vi "Main.vi"(11 "Module Admin":refnum<class "Delacor_lib_QMH_Cloneable Module Admin.lvclass">) -> ()   [LabVIEW 2020, in "NI DAQ Aug 25.lvlib"]
doc: "This template is based off of the Queued Message Handler design pattern and the Queued Message Handler project template that ships with LabVIEW.\n\nThe main difference is that the queue is private to this module and communication between modules is performed via Broadcast and Request events.\n\nRequest events are wrapped in public API methods and are handled in the Event Handling Loop (EHL) of this VI. Any module can register for Broadcast events sent by this module. The EHL generates messages based on user interface actions.\n\nThe Message Handling Loop (MHL) processes messages generated by the EHL, or by other messages. The messages are string values, so new messages can be added easily to the Message Cases case structure in the MHL. Each message cluster can also provide an optional value for Message Data, which is a variant that can be converted to whatever message-specific data is required.\n_____\nBased on DQMH Dev Tools: Project Template 7.1.0.1499."
uses:
  NI DAQ Aug 25.lvlib
  <vilib>/Delacor/Delacor QMH/Libraries/Cloneable Module Admin_class/Delacor_lib_QMH_Cloneable Module Admin.lvclass
  C:/Program Files (x86)/National Instruments/LabVIEW 2025/vi.lib/Delacor/Delacor QMH/Libraries/Module Admin_class/Delacor_lib_QMH_Module Admin.lvclass
  <vilib>/Delacor/Delacor QMH/Libraries/Message Queue_class/Delacor_lib_QMH_Message Queue.lvclass/Delacor_lib_QMH_Message Queue.ctl
  <vilib>/Delacor/Delacor QMH/Libraries/Cloneable Module Admin_class/Delacor_lib_QMH_Cloneable Module Admin.lvclass/Delacor_lib_QMH_Cloneable Module Admin.ctl
  <vilib>/Delacor/Delacor QMH/Libraries/Module Admin_class/Delacor_lib_QMH_Module Admin.lvclass/Delacor_lib_QMH_Module Admin.ctl
  <vilib>/Delacor/Delacor QMH/Libraries/Message Queue_class/Delacor_lib_QMH_Message Queue.lvclass
  Module Data--cluster.ctl
  <vilib>/Utility/miscctls.llb/LVPointTypeDef.ctl
  <vilib>/Delacor/Delacor QMH/Libraries/Message Queue_class/Delacor_lib_QMH_Enqueue Message (Single).vi
  Stop Argument--cluster.ctl
  Draw FP in subpanel Argument--cluster.ctl
  Remove from subpanel Argument--cluster.ctl
  Set device name Argument--cluster.ctl
  <resource>/objmgr/daqmx.rc
  Ports --typedef.ctl
  Write DO Argument--cluster.ctl
  Create DO channel Argument--cluster.ctl
  <vilib>/DAQmx/create/channels.llb/DAQmx Create Channel (DO-Digital Output).vi
  Acquisition type--typedef.ctl
  <vilib>/DAQmx/write.llb/DAQmx Write (Digital Bool 1Line 1Point).vi
  <vilib>/DAQmx/write.llb/DAQmx Write (Digital 1D U8 1Chan NSamp).vi
panel:
  out "error out":errorcluster
  out "Status":string
  in  "Simulate EHL Error":bool
  in  "Simulate MHL Error":bool
  # "Other processes communicate with this Module via its Public API (wrappers for its Request Events).\n\nThis Module communicates with other processes via its Broadcast Events.\nAny process that wants to receive these messages can register for this module's Broadcast events."
  # "This template is for the DQMH framework. See the block diagram for more information on how to use this template."
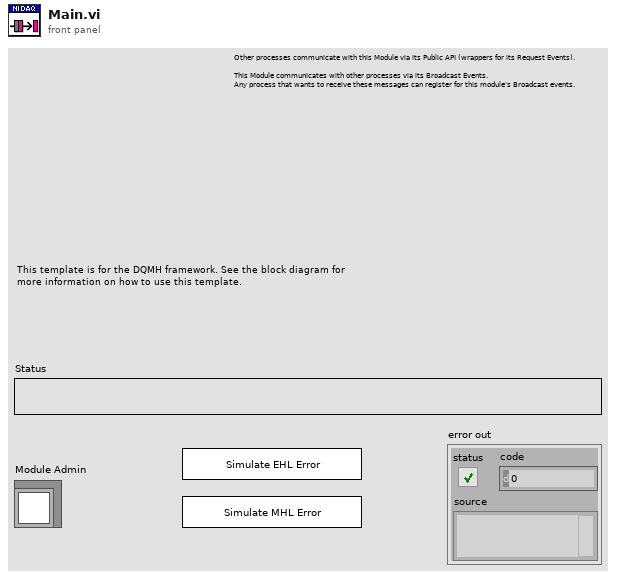
[diagram p1: front panel]
types:
  T1 = typedef "NI DAQ Aug 25.lvlib/Request Events--cluster.ctl" = cluster{"Stop Module":refnum<user-event>, "Show Panel":refnum<user-event>, "Hide Panel":refnum<user-event>, "Show Diagram":refnum<user-event>, "Get Module Execution Status":refnum<user-event>, "Draw FP in subpanel":refnum<user-event>, "Remove from subpanel":refnum<user-event>, "Set device name":refnum<user-event>, "Write DO":refnum<user-event>, "Create DO channel":refnum<user-event>}
  T2 = typedef "NI DAQ Aug 25.lvlib/Module Data--cluster.ctl" = cluster{"Status":string, "Sub Panel":refnum<vi>, "Device Name":tag, "Is simulated?":bool, "DO channel":refnum<k21>}
  T3 = enum32{"invalid lock state", "Not Locked", "Locked (No Password)", "Password-protected"}
  T4 = typedef "NI DAQ Aug 25.lvlib/Stop Argument--cluster.ctl" = cluster{"Module ID":i32, "Origin":string, "Exit via Stop Module Req?":bool, "Wait for Module to stop?":bool}
  T5 = typedef "NI DAQ Aug 25.lvlib/Draw FP in subpanel Argument--cluster.ctl" = cluster{"Module ID":i32, "Sub Panel":refnum<vi>}
  T6 = typedef "NI DAQ Aug 25.lvlib/Remove from subpanel Argument--cluster.ctl" = cluster{"Module ID":i32, "Boolean":bool}
  T7 = typedef "NI DAQ Aug 25.lvlib/Set device name Argument--cluster.ctl" = cluster{"Module ID":i32, "DAQmx Device Name":tag}
  T8 = typedef "NI DAQ Aug 25.lvlib/Write DO Argument--cluster.ctl" = cluster{"Module ID":i32, "Port":T9, "DO":bool[], "Acq type":T10}
  T9 = typedef "Ports --typedef.ctl" = enum16{"port0", "port1"}
  T10 = typedef "Acquisition type--typedef.ctl" = enum16{"Single", "Multiple"}
  T11 = typedef "NI DAQ Aug 25.lvlib/Create DO channel Argument--cluster.ctl" = cluster{"Module ID":i32, "Port":T9, "Lines":string}
  T12 = typedef "LVPointTypeDef.ctl" = cluster{"Horizontal":i16, "Vertical":i16}
  T13 = enum32{"Invalid", "Standard", "Closed", "Hidden", "Minimized", "Maximized"}
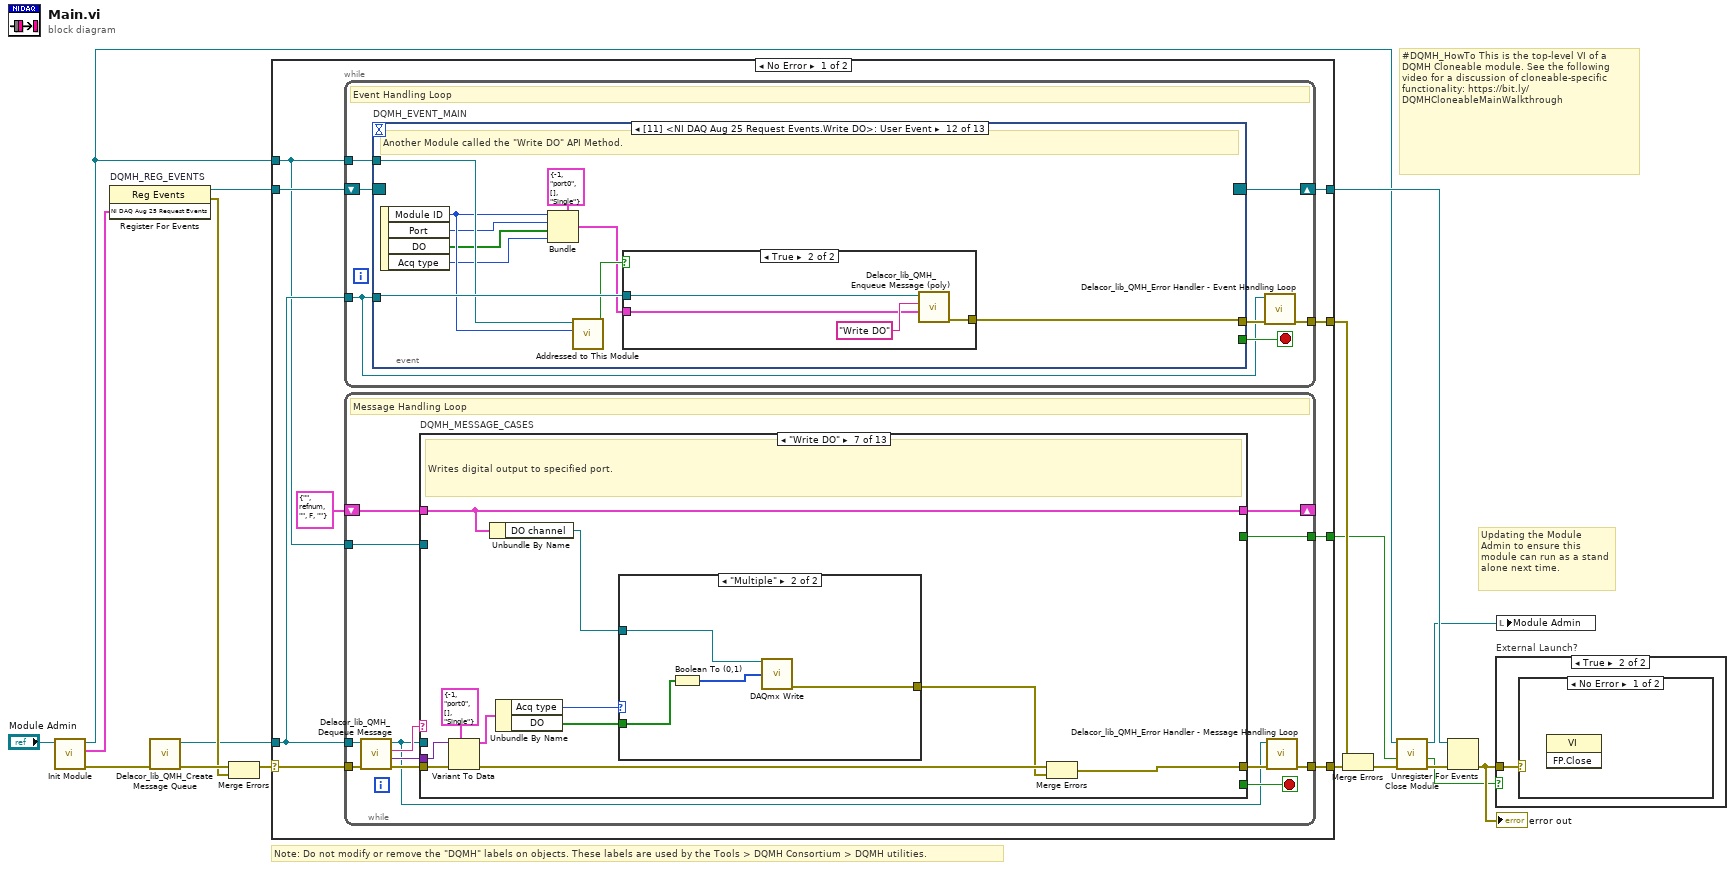
[diagram p0: block diagram]
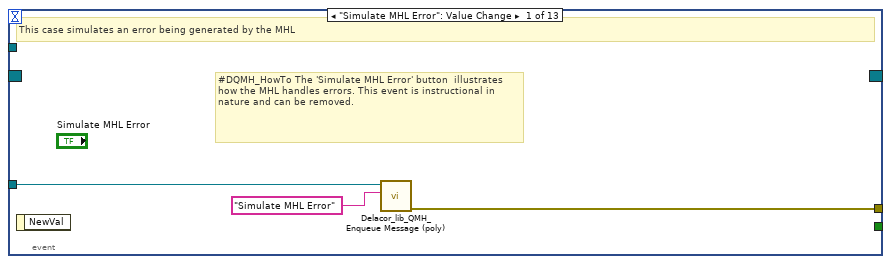
[diagram p2: hidden frame]
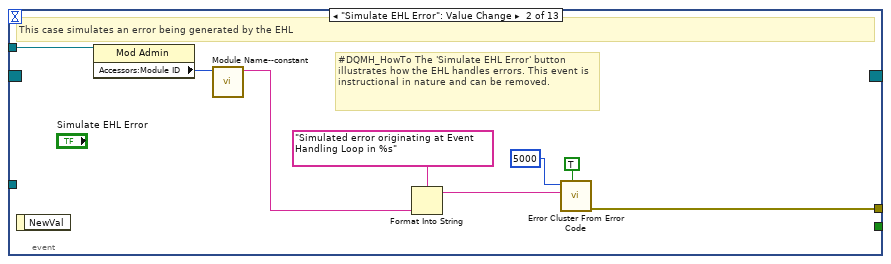
[diagram p3: hidden frame]
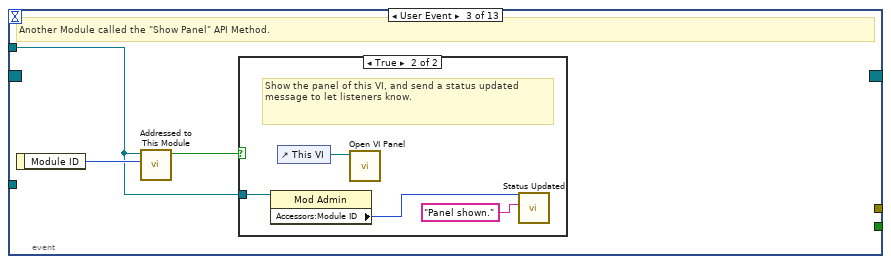
[diagram p4: hidden frame]
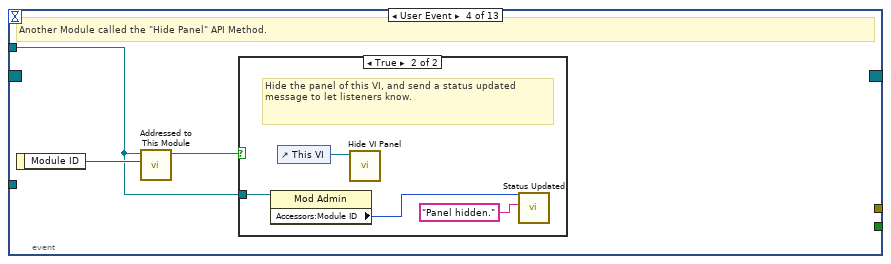
[diagram p6: hidden frame]
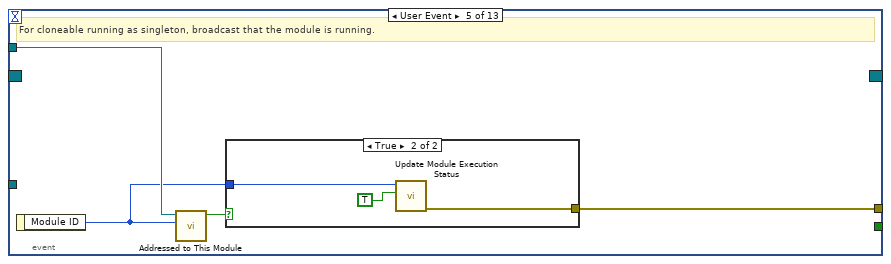
[diagram p8: hidden frame]
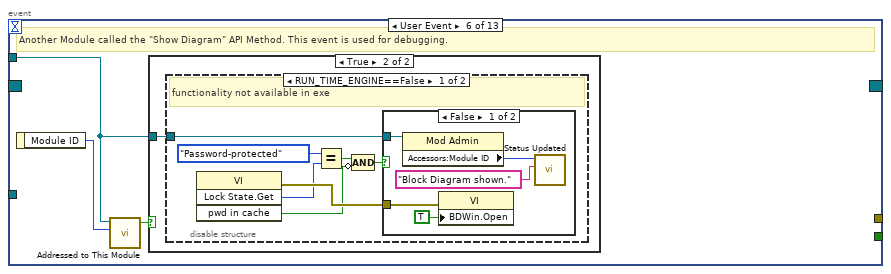
[diagram p10: hidden frame]
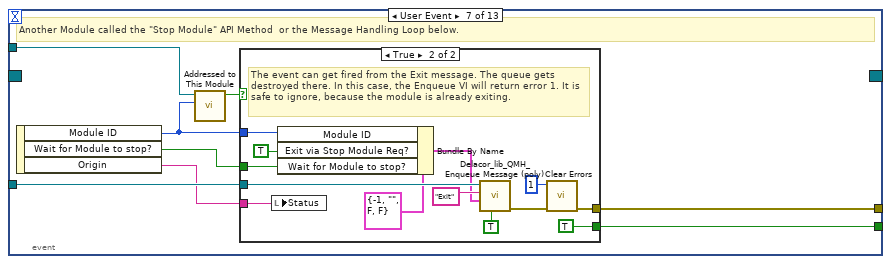
[diagram p14: hidden frame]
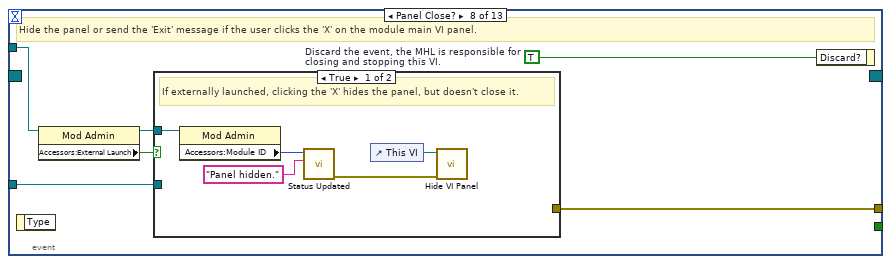
[diagram p16: hidden frame]
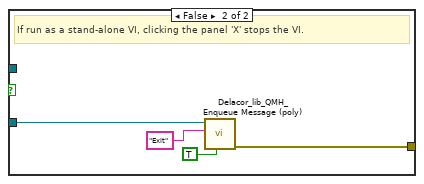
[diagram p17: hidden frame]
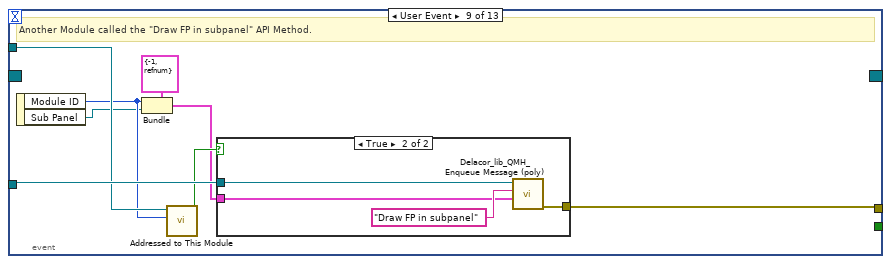
[diagram p18: hidden frame]
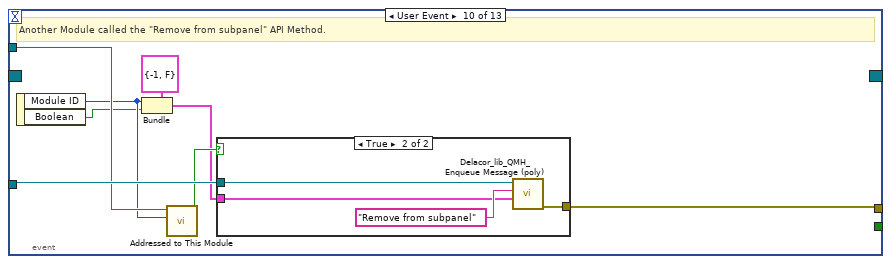
[diagram p20: hidden frame]
diagram:
  # "#DQMH_HowTo This is the top-level VI of a DQMH Cloneable module. See the following video for a discussion of cloneable-specific functionality: https://bit.ly/DQMHCloneableMainWalkthrough"
  # "Note: Do not modify or remove the \"DQMH\" labels on objects. These labels are used by the Tools > DQMH Consortium > DQMH utilities."
  # "Updating the Module Admin to ensure this module can run as a stand alone next time."
  n1 = call "Init Module.vi"("Cloneable Module Admin in"="Module Admin") -> ("error out"=w15:errorcluster, "NI DAQ Aug 25 Request Events"=w7:T1, "Cloneable Module Admin out"=w4:refnum<class "Delacor_lib_QMH_Cloneable Module Admin.lvclass">)  [unwired: 8 in]
  n2 = register-events "DQMH_REG_EVENTS"(w7) -> (reference out=w8:refnum<event-registration>, error out=w10:errorcluster)  [unwired: 2 in]
  n3 = call <vilib>:"Delacor_lib_QMH_Create Message Queue.vi"("error in"=w15) -> ("error out"=w12:errorcluster, "Message Queue"=w6:refnum<class "Delacor_lib_QMH_Message Queue.lvclass">)  [unwired: 9 in]
  n4 = Merge Errors(w12, w10) -> (w11:errorcluster)
  n5 = case shown="No Error" w11 {
    selector: w11 -> [w25 w377]
    tunnel: [w27 w376] -> w16
    tunnel: [w24 w375] -> w9
    tunnel: w8 -> [w22 w375]
    tunnel: w6 -> [w21 w368]
    tunnel: [w26 _] -> w17
    tunnel: w4 -> [w20 w371]
    tunnel: [w19 _] -> w2
    frame No Error {
      n6 = while {
        tunnel: w21 -> [w28]
        shift-right: [w31] -> w24
        shift-left: w22 -> [w32]
        tunnel: [w33] -> w26
        tunnel: w20 -> [w29]
        stop <- w30 stop-if-true
        # "Event Handling Loop"
        n7 = event "DQMH_EVENT_MAIN" shown="[11] <NI DAQ Aug 25 Request Events.Write DO>: User Event" {
          selector: w32 -> [_ _ _ _ _ _ _ _ _ _ _ _ _]
          dyn-events: [_ _ _ _ _ _ _ _ _ _ _ _ _] -> w31
          timeout: _ -> [_ _ _ _ _ _ _ _ _ _ _ _ _]
          tunnel: [_ _ _ _ _ _ w86 _ _ _ _ _ _] -> w30
          tunnel: w28 -> [w36 _ _ _ _ _ w89 w106 w126 w138 w150 w164 w177]
          tunnel: [w37 w45 _ _ w63 _ w90 w109 w119 w131 w143 w156 w169] -> w34
          tunnel: w29 -> [_ w44 w46 w53 w61 w67 w88 w107 w124 w136 w148 w162 w175]
          event "Simulate MHL Error": Value Change {
            # "#DQMH_HowTo The 'Simulate MHL Error' button  illustrates how the MHL handles errors. This event is instructional in nature and can be removed."
            # "This case simulates an error being generated by the MHL"
            n8 = event-data() -> ()  [unwired: 1 in, 1 out]
            n9 = call-poly <vilib>:"Delacor_lib_QMH_Enqueue Message (poly).vi"("Message"="Simulate MHL Error", "Message Queue in"=w36) -> ("error out"=w37:errorcluster)  [unwired: 8 in, 1 out]
          }
          event "Simulate EHL Error": Value Change {
            # "#DQMH_HowTo The 'Simulate EHL Error' button  illustrates how the EHL handles errors. This event is instructional in nature and can be removed."
            # "This case simulates an error being generated by the EHL"
            n10 = event-data() -> ()  [unwired: 1 in, 1 out]
            n11 = property on="Property Node" class="Mod Admin"(reference=w44) -> ("Accessors:Module ID"=w43:i32)  [unwired: 1 in, 2 out]
            n12 = call "Module Name--constant.vi"("Module ID"=w43) -> ("Module Name"=w38:string)  [unwired: 10 in]
            n13 = Format Into String(format string="Simulated error originating at Event Handling Loop in %s", w38) -> (resulting string=w41:string)  [unwired: 2 in, 1 out]
            n14 = call <vilib>:"Error Cluster From Error Code.vi"("show call chain? (False)"=TRUE, "error message (\"\")"=w41, "error code (0)"=5000) -> ("error out"=w45:errorcluster)  [unwired: 6 in]
          }
          event User Event {
            # "Another Module called the \"Show Panel\" API Method."
            n15 = event-data() -> ("Module ID"=w47:i32)  [unwired: 1 in]
            n16 = call "Addressed to This Module.vi"("Module ID from Argument"=w47, "Module Admin"=w46) -> ("Addressed to this instance?"=w48:bool)  [unwired: 8 in, 1 out]
            n17 = case shown="True" w48 {
              tunnel: w46 -> [_ w50]
              frame False {
              }
              frame True {
                # "Show the panel of this VI, and send a status updated message to let listeners know."
                n18 = property on="Property Node" class="Mod Admin"(reference=w50) -> ("Accessors:Module ID"=w49:i32)  [unwired: 1 in, 2 out]
                n19 = control-ref of="This VI"() -> (w52:refnum<vi>)
                n20 = call "Open VI Panel.vi"("VI"=w52) -> ()  [unwired: 10 in, 1 out]
                n21 = call "Status Updated.vi"("Status"="Panel shown." ("format string"), "Module ID"=w49) -> ()  [unwired: 9 in, 1 out]
              }
            }
          }
          event User Event {
            # "Another Module called the \"Hide Panel\" API Method."
            n22 = event-data() -> ("Module ID"=w54:i32)  [unwired: 1 in]
            n23 = call "Addressed to This Module.vi"("Module ID from Argument"=w54, "Module Admin"=w53) -> ("Addressed to this instance?"=w55:bool)  [unwired: 8 in, 1 out]
            n24 = case shown="True" w55 {
              tunnel: w53 -> [_ w57]
              frame False {
              }
              frame True {
                # "Hide the panel of this VI, and send a status updated message to let listeners know."
                n25 = property on="Property Node" class="Mod Admin"(reference=w57) -> ("Accessors:Module ID"=w56:i32)  [unwired: 1 in, 2 out]
                n26 = control-ref of="This VI"() -> (w59:refnum<vi>)
                n27 = call "Hide VI Panel.vi"("VI"=w59) -> ()  [unwired: 10 in, 1 out]
                n28 = call "Status Updated.vi"("Status"="Panel hidden." ("format string"), "Module ID"=w56) -> ()  [unwired: 9 in, 1 out]
              }
            }
          }
          event User Event {
            # "For cloneable running as singleton, broadcast that the module is running."
            n29 = event-data() -> ("Module ID"=w60:i32)  [unwired: 1 in]
            n30 = call "Addressed to This Module.vi"("Module ID from Argument"=w60, "Module Admin"=w61) -> ("Addressed to this instance?"=w62:bool)  [unwired: 8 in, 1 out]
            n31 = case shown="True" w62 {
              tunnel: [_ w66] -> w63
              tunnel: w60 -> [_ w65]
              frame False {
              }
              frame True {
                n32 = call "Update Module Execution Status.vi"("Running?"=TRUE, "Module ID"=w65) -> ("error out"=w66:errorcluster)  [unwired: 9 in]
              }
            }
          }
          event User Event {
            # "Another Module called the \"Show Diagram\" API Method. This event is used for debugging."
            n33 = event-data() -> ("Module ID"=w68:i32)  [unwired: 1 in]
            n34 = call "Addressed to This Module.vi"("Module ID from Argument"=w68, "Module Admin"=w67) -> ("Addressed to this instance?"=w69:bool)  [unwired: 8 in, 1 out]
            n35 = case shown="True" w69 {
              tunnel: w67 -> [_ w70]
              frame False {
              }
              frame True {
                n36 = disable-structure shown="RUN_TIME_ENGINE==False" {
                  disable-tunnel: w70 -> [w71 _]
                  frame condition #0 (active) {
                    # "functionality not available in exe"
                    n37 = invoke on="Invoke Node" class="VI" method="Lock State.Get"() -> (error out=w77:errorcluster, "Get Lock State"=w76:T3, "pwd in cache"=w73:bool)  [unwired: 4 in, 1 out]
                    n38 = Equal?(x=T3."Password-protected", y=w76) -> (x = y?=w74:bool)
                    n39 = Compound Arithmetic op=AND(w74, invert w73) -> (w72:bool)
                    n40 = case shown="False" w72 {
                      tunnel: w77 -> [w82 _]
                      tunnel: w71 -> [w79 _]
                      frame False {
                        n41 = property on="Property Node" class="Mod Admin"(reference=w79) -> ("Accessors:Module ID"=w78:i32)  [unwired: 1 in, 2 out]
                        n42 = property on="Property Node" class="VI"(error in=w82, "BDWin.Open"=TRUE ("Block Diagram Window:Open")) -> ()  [unwired: 1 in, 2 out]
                        n43 = call "Status Updated.vi"("Status"="Block Diagram shown." ("format string"), "Module ID"=w78) -> ()  [unwired: 9 in, 1 out]
                      }
                      frame True {
                        # "Password-protected VI, and the password is not in the cache. Do not show the diagram."
                      }
                    }
                  }
                  frame condition #1 {
                  }
                }
              }
            }
          }
          event User Event {
            # "Another Module called the \"Stop Module\" API Method  or the Message Handling Loop below."
            n44 = event-data() -> ("Module ID"=w84:i32, "Wait for Module to stop?"=w85:bool, "Origin"=w83:string)  [unwired: 1 in]
            n45 = call "Addressed to This Module.vi"("Module ID from Argument"=w84, "Module Admin"=w88) -> ("Addressed to this instance?"=w87:bool)  [unwired: 8 in, 1 out]
            n46 = case shown="True" w87 {
              tunnel: [_ w102] -> w90
              tunnel: w89 -> [_ w98]
              tunnel: [_ TRUE] -> w86
              tunnel: w85 -> [_ w93]
              tunnel: w84 -> [_ w95]
              tunnel: w83 -> [_ w91]
              frame False {
              }
              frame True {
                # "The event can get fired from the Exit message. The queue gets destroyed there. In this case, the Enqueue VI will return error 1. It is safe to ignore, because the module is already exiting."
                n47 = local write "Status"(w91) -> ()
                n48 = Bundle By Name(cluster=T4 {"Module ID"=-1, "Origin"="", "Exit via Stop Module Req?"=FALSE, "Wait for Module to stop?"=FALSE} ("Stop Argument"), "Module ID"=w95, "Exit via Stop Module Req?"=TRUE, "Wait for Module to stop?"=w93) -> (w92:T4)
                n49 = call-poly <vilib>:"Delacor_lib_QMH_Enqueue Message (poly).vi"("Priority Message? (F)"=TRUE, "Message Data"=w92, "Message"="Exit", "Message Queue in"=w98) -> ("error out"=w103:errorcluster)  [unwired: 6 in, 1 out]
                n50 = call <vilib>:"Clear Errors.vi"("error in (no error)"=w103, "specific error code to clear (0: all)"=1) -> ("error out"=w102:errorcluster)  [unwired: 4 in, 1 out]
              }
            }
          }
          event Panel Close? {
            w108 = TRUE  # Discard the event, the MHL is responsible for closing and stopping this VI.
            # "Hide the panel or send the 'Exit' message if the user clicks the 'X' on the module main VI panel."
            n51 = event-data() -> ()  [unwired: 1 in, 1 out]
            n52 = property on="Property Node" class="Mod Admin"(reference=w107) -> (reference out=w104:refnum<class "Delacor_lib_QMH_Cloneable Module Admin.lvclass">, "Accessors:External Launch"=w105:bool)  [unwired: 1 in, 1 out]
            n53 = case shown="True" w105 {
              tunnel: w106 -> [_ w117]
              tunnel: [_ w118] -> w109
              tunnel: w104 -> [w112 _]
              frame True {
                # "If externally launched, clicking the 'X' hides the panel, but doesn't close it."
                n54 = property on="Property Node" class="Mod Admin"(reference=w112) -> ("Accessors:Module ID"=w111:i32)  [unwired: 1 in, 2 out]
                n55 = call "Status Updated.vi"("Status"="Panel hidden." ("format string"), "Module ID"=w111) -> ("error out"=w110:errorcluster)  [unwired: 9 in]
                n56 = control-ref of="This VI"() -> (w114:refnum<vi>)
                n57 = call "Hide VI Panel.vi"("error in"=w110, "VI"=w114) -> ()  [unwired: 9 in, 1 out]
              }
              frame False {
                # "If run as a stand-alone VI, clicking the panel 'X' stops the VI."
                n58 = call-poly <vilib>:"Delacor_lib_QMH_Enqueue Message (poly).vi"("Priority Message? (F)"=TRUE, "Message"="Exit", "Message Queue in"=w117) -> ("error out"=w118:errorcluster)  [unwired: 7 in, 1 out]
              }
            }
            n59 = event-data ("Event Filter Node")("Discard?"=w108) -> ()  [unwired: 1 in, 1 out]
          }
          event User Event {
            # "Another Module called the \"Draw FP in subpanel\" API Method."
            n60 = event-data() -> ("Module ID"=w121:i32, "Sub Panel"=w120:refnum<vi>)  [unwired: 1 in]
            n61 = Bundle(cluster=T5 {"Module ID"=-1, "Sub Panel"=refnum} ("Draw FP in subpanel Argument"), "Module ID"=w121, "Sub Panel"=w120) -> (w122:T5)
            n62 = call "Addressed to This Module.vi"("Module ID from Argument"=w121, "Module Admin"=w124) -> ("Addressed to this instance?"=w125:bool)  [unwired: 8 in, 1 out]
            n63 = case shown="True" w125 {
              tunnel: w126 -> [_ w130]
              tunnel: w122 -> [_ w128]
              tunnel: [_ w127] -> w119
              frame False {
              }
              frame True {
                n64 = call-poly <vilib>:"Delacor_lib_QMH_Enqueue Message (poly).vi"("Message Data"=w128, "Message"="Draw FP in subpanel", "Message Queue in"=w130) -> ("error out"=w127:errorcluster)  [unwired: 7 in, 1 out]
              }
            }
          }
          event User Event {
            # "Another Module called the \"Remove from subpanel\" API Method."
            n65 = event-data() -> ("Module ID"=w133:i32, "Boolean"=w132:bool)  [unwired: 1 in]
            n66 = Bundle(cluster=T6 {"Module ID"=-1, "Boolean"=FALSE} ("Remove from subpanel Argument"), "Module ID"=w133, "Boolean"=w132) -> (w134:T6)
            n67 = call "Addressed to This Module.vi"("Module ID from Argument"=w133, "Module Admin"=w136) -> ("Addressed to this instance?"=w137:bool)  [unwired: 8 in, 1 out]
            n68 = case shown="True" w137 {
              tunnel: w138 -> [_ w142]
              tunnel: w134 -> [_ w140]
              tunnel: [_ w139] -> w131
              frame False {
              }
              frame True {
                n69 = call-poly <vilib>:"Delacor_lib_QMH_Enqueue Message (poly).vi"("Message Data"=w140, "Message"="Remove from subpanel", "Message Queue in"=w142) -> ("error out"=w139:errorcluster)  [unwired: 7 in, 1 out]
              }
            }
          }
          event User Event {
            # "Another Module called the \"Set device name\" API Method."
            n70 = event-data() -> ("Module ID"=w145:i32, "DAQmx Device Name"=w144:tag)  [unwired: 1 in]
            n71 = Bundle(cluster=T7 {"Module ID"=-1, "DAQmx Device Name"=""} ("Set device name Argument"), "Module ID"=w145, "DAQmx Device Name"=w144) -> (w146:T7)
            n72 = call "Addressed to This Module.vi"("Module ID from Argument"=w145, "Module Admin"=w148) -> ("Addressed to this instance?"=w149:bool)  [unwired: 8 in, 1 out]
            n73 = case shown="True" w149 {
              tunnel: w150 -> [_ w154]
              tunnel: w146 -> [_ w152]
              tunnel: [_ w151] -> w143
              frame False {
              }
              frame True {
                n74 = call-poly <vilib>:"Delacor_lib_QMH_Enqueue Message (poly).vi"("Message Data"=w152, "Message"="Set device name", "Message Queue in"=w154) -> ("error out"=w151:errorcluster)  [unwired: 7 in, 1 out]
              }
            }
          }
          event User Event {
            # "Another Module called the \"Write DO\" API Method."
            n75 = event-data() -> ("Module ID"=w159:i32, "Port"=w158:T9, "DO"=w157:bool[], "Acq type"=w155:T10)  [unwired: 1 in]
            n76 = Bundle(cluster=T8 {"Module ID"=-1, "Port"=enum."port0", "DO"=[], "Acq type"=enum."Single"} ("Write DO Argument"), "Module ID"=w159, "Port"=w158, "DO"=w157, "Acq type"=w155) -> (w160:T8)
            n77 = call "Addressed to This Module.vi"("Module ID from Argument"=w159, "Module Admin"=w162) -> ("Addressed to this instance?"=w163:bool)  [unwired: 8 in, 1 out]
            n78 = case shown="True" w163 {
              tunnel: w164 -> [_ w168]
              tunnel: w160 -> [_ w166]
              tunnel: [_ w165] -> w156
              frame False {
              }
              frame True {
                n79 = call-poly <vilib>:"Delacor_lib_QMH_Enqueue Message (poly).vi"("Message Data"=w166, "Message"="Write DO", "Message Queue in"=w168) -> ("error out"=w165:errorcluster)  [unwired: 7 in, 1 out]
              }
            }
          }
          event User Event {
            # "Another Module called the \"Create DO channel\" API Method."
            n80 = event-data() -> ("Module ID"=w172:i32, "Port"=w171:T9, "Lines"=w170:string)  [unwired: 1 in]
            n81 = Bundle(cluster=T11 {"Module ID"=-1, "Port"=enum."port0", "Lines"=""} ("Create DO channel Argument"), "Module ID"=w172, "Port"=w171, "Lines"=w170) -> (w173:T11)
            n82 = call "Addressed to This Module.vi"("Module ID from Argument"=w172, "Module Admin"=w175) -> ("Addressed to this instance?"=w176:bool)  [unwired: 8 in, 1 out]
            n83 = case shown="True" w176 {
              tunnel: w177 -> [_ w181]
              tunnel: w173 -> [_ w179]
              tunnel: [_ w178] -> w169
              frame False {
              }
              frame True {
                n84 = call-poly <vilib>:"Delacor_lib_QMH_Enqueue Message (poly).vi"("Message Data"=w179, "Message"="Create DO channel", "Message Queue in"=w181) -> ("error out"=w178:errorcluster)  [unwired: 7 in, 1 out]
              }
            }
          }
        }
        n85 = call-dynamic "Delacor_lib_QMH_Error Handler - Event Handling Loop.vi"("error in"=w34, "Message Queue in"=w28) -> ("dup error in"=w33:errorcluster)  [unwired: 8 in, 1 out]
      }
      n86 = while {
        tunnel: w21 -> [w182]
        shift-right: [w189] -> _
        shift-left: T2 {"Status"="", "Sub Panel"=refnum, "Device Name"="", "Is simulated?"=FALSE, "DO channel"=""} ("Data Cluster") -> [w190]
        tunnel: w25 -> [w193]
        tunnel: [w191] -> w27
        tunnel: w20 -> [w184]
        tunnel: [w183] -> w19
        stop <- w188 stop-if-true
        # "Message Handling Loop"
        n87 = call-dynamic "Delacor_lib_QMH_Dequeue Message.vi"("error in"=w193, "Message Queue in"=w182) -> ("error out"=w192:errorcluster, "Message Data"=w186:variant, "Message"=w187:string, "Message Queue out"=w185:refnum<class "Delacor_lib_QMH_Message Queue.lvclass">)  [unwired: 6 in]
        n88 = case "DQMH_MESSAGE_CASES" shown="\"Write DO\"" w187 {
          selector: w187 -> [_ _ _ _ _ _ _ _ _ _ _ _ w357]
          tunnel: w185 -> [_ _ _ _ _ _ _ _ _ w311 _ w349 _]
          tunnel: w192 -> [w213 w217 w231 w243 w266 w284 w295 w306 w308 w320 w337 w355 w366]
          tunnel: [w211 w217 w230 w235 w262 w271 w286 w305 w308 w316 w336 w350 w367] -> w194
          tunnel: w190 -> [w204 w216 w222 w236 w255 w273 w289 w304 w307 w315 w334 w339 w364]
          tunnel: [w203 w216 w221 w236 w253 w272 w289 w304 w307 w315 w334 w339 w364] -> w189
          tunnel: [_ _ _ _ _ _ _ _ _ _ _ w348 _] -> w188
          tunnel: w186 -> [_ _ w229 w241 w265 w282 w293 _ _ w314 _ w346 _]
          tunnel: w184 -> [w199 _ _ w233 w252 _ _ _ _ w313 w332 w341 w363]
          tunnel: [_ _ _ _ _ _ _ _ _ _ _ w344 _] -> w183
          frame "Initialize" {
            w196 = "Initial Message" ("Initial Message")
            # "#DQMH_CodeNeeded - Initialize the appearance of the front panel."
            # "#DQMH_CodeNeeded - Initialize your state data here."
            # "Initialize - Any operation that needs to be done before the module can receive messages. Synchronize Caller Events.vi will inform Start Module.vi that the module has launched and is ready to receive messages. Module Did Init.vi will broadcast that the module initialized."
            n89 = call "Synchronize Caller Events.vi"("error in"=w213, "Module Admin"=w199) -> ("error out"=w212:errorcluster, "Module Admin out"=w198:refnum<class "Delacor_lib_QMH_Cloneable Module Admin.lvclass">)  [unwired: 8 in]
            n90 = property on="Property Node" class="Mod Admin"(reference=w198) -> ("Accessors:Module ID"=w195:i32, "Accessors:External Launch"=w200:bool)  [unwired: 1 in, 2 out]
            n91 = call "Module Name--constant.vi"("Module ID"=w195) -> ("Module Name"=w208:string)  [unwired: 10 in]
            n92 = property on="Property Node" class="VI"("Front Panel.Title"=w208) -> (reference out=w210:refnum<vi>, error out=w215:errorcluster)  [unwired: 2 in]
            n93 = Select(t=T13."Hidden" ("State"), s=w200, f=T13."Standard" ("State")) -> (s? t:f=w205:T13)
            n94 = invoke on="Invoke Node" class="VI" method="FP.Open"(reference=w210, error in=w215, "State"=w205) -> (reference out=w209:refnum<vi>, error out=w214:errorcluster)  [unwired: 2 in, 3 out]
            n95 = Bundle By Name(cluster=w204, "Status"=w196) -> (w203:T2)
            n96 = invoke on="Invoke Node" class="VI" method="FP.Center"(reference=w209, error in=w214) -> ()  [unwired: 1 in, 3 out]
            n97 = property on="Pane" class="Pane"("Origin"=T12 {"Horizontal"=0, "Vertical"=0}) -> ()  [unwired: 2 in, 2 out]
            n98 = call "Module Name--constant.vi"("Module ID"=w195) -> ("Module Name"=w201:string)  [unwired: 10 in]
            n99 = call "Module Did Init.vi"("error in"=w212, "Initialized?"=TRUE, "Origin"=w201, "Module ID"=w195) -> ("error out"=w211:errorcluster)  [unwired: 7 in]
            "Status" <- w196
          }
          frame "---Module Specific---" {
            # "Separator -- The following cases handle messages specific to this Module."
          }
          frame "Draw FP in subpanel" {
            # "The VI cannot be inserted in a subpanel because VI is already opened."
            # "Draw FP in subpanel"
            n100 = Variant To Data(error in=w231, type=T5 {"Module ID"=-1, "Sub Panel"=refnum} ("Draw FP in subpanel Argument"), Variant=w229) -> (data=w227:T5, error out=w230:errorcluster)
            n101 = Unbundle By Name(w227) -> ("Sub Panel"=w220:refnum<vi>)  [unwired: 1 out]
            n102 = control-ref of="This VI"() -> (w226:refnum<vi>)
            n103 = invoke class="VI" method="FP.Close"(reference=w226) -> (reference out=w219:refnum<vi>, error out=w225:errorcluster)  [unwired: 2 in, 1 out]
            n104 = call <vilib>:"Clear Errors.vi"("error in (no error)"=w225, "specific error code to clear (0: all)"=1144) -> ("error out"=w224:errorcluster)  [unwired: 4 in, 1 out]
            n105 = invoke class="SubPnl" method="Insert VI"(reference=w220, error in=w224, "VI Ref"=w219) -> (reference out=w218:refnum<vi>)  [unwired: 1 in, 3 out]
            n106 = Bundle By Name(cluster=w222, "Sub Panel"=w218) -> (w221:T2)
          }
          frame "Remove from subpanel" {
            # "Remove panel from subpanel"
            n107 = property class="Mod Admin"(reference=w233) -> ("Accessors:Module ID"=w232:i32)  [unwired: 1 in, 2 out]
            n108 = Variant To Data(error in=w243, type=T6 {"Module ID"=-1, "Boolean"=FALSE} ("Remove from subpanel Argument"), Variant=w241) -> (data=w239:T6, error out=w242:errorcluster)
            n109 = Unbundle By Name(w239) -> ()  [unwired: 2 out]
            n110 = Unbundle By Name(w236) -> ("Sub Panel"=w237:refnum<vi>)
            n111 = Not A Number/Path/Refnum?(number/path/refnum=w237) -> (NaN/Path/Refnum?=w238:bool)
            n112 = case shown="True" w238 {
              tunnel: w237 -> [w245 _]
              tunnel: [w244 _] -> w234
              tunnel: w232 -> [_ w247]
              frame False {
                n113 = invoke class="SubPnl" method="Remove VI"(reference=w245) -> (error out=w244:errorcluster)  [unwired: 2 in, 2 out]
              }
              frame True {
                n114 = call "Status Updated.vi"("Status"="Subpanel reference is null. Call Draw in FP first.", "Module ID"=w247) -> ()  [unwired: 9 in, 1 out]
              }
            }
            n115 = Merge Errors(w242, w234) -> (w235:errorcluster)
          }
          frame "Set device name" {
            # "Sets selected device name to private data cluster."
            n116 = Variant To Data(error in=w266, type=T7 {"Module ID"=-1, "DAQmx Device Name"=""} ("Set device name Argument"), Variant=w265) -> (data=w263:T7, error out=w261:errorcluster)
            n117 = Unbundle By Name(w263) -> ("DAQmx Device Name"=w249:tag)  [unwired: 1 out]
            n118 = property class="Mod Admin"(reference=w252) -> ("Accessors:Module ID"=w251:i32)  [unwired: 1 in, 2 out]
            n119 = property class="DAQmx Device"(error in=w261, "Active Device"=w249) -> (error out=w262:errorcluster, "ProductType"=w259:string, "DevIsSimulated"=w254:bool)  [unwired: 1 in, 1 out]
            n120 = Bundle By Name(cluster=w255, "Device Name"=w249, "Is simulated?"=w254) -> (w253:T2)
            n121 = Select(t="simulated" ("format string"), s=w254, f="physical device") -> (s? t:f=w256:string)
            n122 = call "Get channels list.vi"("ActiveDev"=w249) -> ("Channel list"=w248:tag[][])  [unwired: 9 in, 1 out]
            n123 = Format Into String(format string="Active device: %s is %s.", w259, w256) -> (resulting string=w250:string)  [unwired: 2 in, 1 out]
            n124 = call "Device name set.vi"("Channel list"=w248, "Message"=w250, "Module ID"=w251) -> ()  [unwired: 8 in, 1 out]
          }
          frame "Create DO channel" {
            # "Creates a digital output channel with a a single or multiple lines."
            n125 = Variant To Data(error in=w284, type=T11 {"Module ID"=-1, "Port"=enum."port0", "Lines"=""} ("Create DO channel Argument"), Variant=w282) -> (data=w280:T11, error out=w283:errorcluster)
            n126 = Unbundle By Name(w280) -> ("Port"=w277:T9, "Lines"=w276:string)  [unwired: 1 out]
            n127 = Unbundle By Name(w273) -> ("Device Name"=w278:tag)
            n128 = Format Into String(format string="%s/%s/line%s", w278, w277, w276) -> (resulting string=w275:string)  [unwired: 2 in, 1 out]
            n129 = call-poly <vilib>:"DAQmx Create Virtual Channel.vi"("lines"=w275, "name to assign"="DO") -> ("task out"=w268:refnum<k21>, "error out"=w270:errorcluster)  [unwired: 12 in]
            n130 = call <vilib>:"DAQmx Start Task.vi"("task/channels in"=w268, "error in"=w270) -> ("task out"=w267:refnum<k21>, "error out"=w269:errorcluster)  [unwired: 12 in]
            n131 = Bundle By Name(cluster=w273, "DO channel"=w267) -> (w272:T2)
            n132 = Merge Errors(w283, w269) -> (w271:errorcluster)
          }
          frame "Write DO" {
            # "Writes digital output to specified port."
            n133 = Variant To Data(error in=w295, type=T8 {"Module ID"=-1, "Port"=enum."port0", "DO"=[], "Acq type"=enum."Single"} ("Write DO Argument"), Variant=w293) -> (data=w291:T8, error out=w294:errorcluster)
            n134 = Unbundle By Name(w289) -> ("DO channel"=w288:refnum<k21>)
            n135 = Unbundle By Name(w291) -> ("Acq type"=w290:T10, "DO"=w287:bool[])
            n136 = case shown="\"Multiple\"" w290 {
              tunnel: w288 -> [w298 w303]
              tunnel: w287 -> [w297 w301]
              tunnel: [w299 w302] -> w285
              frame "Single", Default {
                n137 = Index Array(array=w297) -> (element=w296:bool)  [unwired: 1 in]
                n138 = call-poly <vilib>:"DAQmx Write.vi"("task/channels in"=w298, "data"=w296) -> ("error out"=w299:errorcluster)  [unwired: 11 in, 2 out]
              }
              frame "Multiple" {
                n139 = Boolean To (0,1)(Boolean=w301) -> (0, 1=w300:i16[])
                n140 = call-poly <vilib>:"DAQmx Write.vi"("task/channels in"=w303, "data"=w300) -> ("error out"=w302:errorcluster)  [unwired: 11 in, 2 out]
              }
            }
            n141 = Merge Errors(w294, w285) -> (w286:errorcluster)
          }
          frame "---Copy This Frame---" {
            # "Duplicate this frame when creating new messages.  Change this comment in the duplicated frame to describe this message."
            n142 = Merge Errors(w306) -> (w305:errorcluster)
          }
          frame "---Exit and Error Handling---" {
            # "Separator - the following cases handle errors and exit messages."
          }
          frame "Error" {
            # "#DQMH_CodeRecommended - If the module is running in standalone mode (External Launch = FALSE), this code will pop up an error dialog and call the 'Exit' message if an error occurs. Add more fine-grained error management here."
            # "Error - Check the error message data and respond accordingly. This message is sent by the \"Error Handler\" VIs at the end of each loop in this application."
            n143 = property on="Property Node" class="Mod Admin"(reference=w313) -> ("Accessors:External Launch"=w312:bool, "Accessors:Module ID"=w310:i32)  [unwired: 1 in, 2 out]
            n144 = Variant To Data(error in=w320, type=errorcluster {"status"=FALSE, "code"=0, "source"=""} ("error constant"), Variant=w314) -> (data=w309:errorcluster, error out=w318:errorcluster)
            n145 = local write "error out"(w309) -> ()
            n146 = call "Error Reported.vi"("Error"=w309, "Module ID"=w310) -> ()  [unwired: 9 in, 1 out]
            n147 = case shown="False" w312 {
              tunnel: [w325 _] -> w317
              tunnel: w311 -> [w323 _]
              tunnel: w309 -> [w324 _]
              frame False {
                n148 = disable-structure shown="Default" {
                  disable-tunnel: w324 -> [w326 _]
                  frame condition #0 (active) {
                    # "If the module is running standalone, then pop up an error dialog and call the \"Exit\" message."
                    n149 = call <vilib>:"Simple Error Handler.vi"("error in (no error)"=w326) -> ()  [unwired: 4 in, 5 out]
                  }
                  frame condition #1 {
                    # "To prevent the Simple Error Handler VI from being loaded (e.g. when deploying to a Real-Time target), add the Conditional Disable Symbol \"DQMH_Disable_SEH\" to your project and set it to TRUE."
                  }
                }
                n150 = call-poly <vilib>:"Delacor_lib_QMH_Enqueue Message (poly).vi"("Priority Message? (F)"=TRUE, "Message"="Exit", "Message Queue in"=w323) -> ("error out"=w325:errorcluster)  [unwired: 7 in, 1 out]
              }
              frame True {
                # "If the module was launched externally, calling the Error Reported broadcast VI is the only action performed by the \"Error\" message. The module's caller can then process the error appropriately."
              }
            }
            n151 = Merge Errors(w318, w317) -> (w316:errorcluster)
          }
          frame "Simulate MHL Error" {
            # "#DQMH_HowTo The 'Simulate MHL Error' button  illustrates how the MHL handles errors. This event is instructional in nature and can be removed."
            # "Simulate an error occurring at the MHL"
            n152 = property on="Property Node" class="Mod Admin"(reference=w332) -> ("Accessors:Module ID"=w333:i32)  [unwired: 1 in, 2 out]
            n153 = call "Module Name--constant.vi"("Module ID"=w333) -> ("Module Name"=w328:string)  [unwired: 10 in]
            n154 = Format Into String(format string="Simulated error originating at Message Handling Loop in %s", w328) -> (resulting string=w329:string)  [unwired: 2 in, 1 out]
            n155 = call <vilib>:"Error Cluster From Error Code.vi"("show call chain? (False)"=TRUE, "error message (\"\")"=w329, "error code (0)"=5001) -> ("error out"=w335:errorcluster)  [unwired: 6 in]
            n156 = Merge Errors(w337, w335) -> (w336:errorcluster)
          }
          frame "Exit" {
            w347 = 91  # 91: not all Exit messages will have an argument
            w348 = TRUE  # Stop the VI
            # "Release the message queue reference"
            # "#DQMH_CodeNeeded - Add any required cleanup code here."
            # "Exit - Exit the application."
            n157 = Variant To Data(error in=w355, type=T4 {"Module ID"=-1, "Origin"="", "Exit via Stop Module Req?"=FALSE, "Wait for Module to stop?"=FALSE} ("Stop Argument"), Variant=w346) -> (data=w343:T4, error out=w351:errorcluster)
            n158 = call <vilib>:"Clear Errors.vi"("error in (no error)"=w351, "specific error code to clear (0: all)"=w347) -> ("error out"=w354:errorcluster)  [unwired: 4 in, 1 out]
            n159 = property on="Property Node" class="Mod Admin"(reference=w341) -> ("Accessors:Module ID"=w340:i32)  [unwired: 1 in, 2 out]
            n160 = control-ref of="This VI"() -> (w342:refnum<vi>)
            n161 = call-dynamic "Delacor_lib_QMH_Release Message Queue.vi"("error in"=w354, "Message Queue"=w349) -> ("error out"=w353:errorcluster)  [unwired: 9 in]
            n162 = call "Handle Exit.vi"("Stop Argument"=w343, "Module Admin in"=w341, "VI reference"=w342) -> ("error out"=w352:errorcluster, "Wait for Stop?"=w344:bool)  [unwired: 7 in]
            n163 = Merge Errors(w353, w352) -> (w350:errorcluster)
            n164 = call "Error Reported.vi"("Error"=w350, "Module ID"=w340) -> ()  [unwired: 9 in, 1 out]
            n165 = Unbundle By Name(w339) -> ("Sub Panel"=w338:refnum<vi>)
            n166 = invoke class="SubPnl" method="Remove VI"(reference=w338) -> ()  [unwired: 2 in, 3 out]
          }
          frame Default {
            # "'Default' case only runs if there is a message that isn't defined in any of the other cases.  Output a programming error."
            n167 = property on="Property Node" class="Mod Admin"(reference=w363) -> ("Accessors:Module ID"=w362:i32)  [unwired: 1 in, 2 out]
            n168 = call "Module Name--constant.vi"("Module ID"=w362) -> ("Module Name"=w356:string)  [unwired: 10 in]
            n169 = Format Into String(format string="The invalid message string \"%s\" was received in the Message Handling Loop for module \"%s\".", w357, w356) -> (resulting string=w359:string)  [unwired: 2 in, 1 out]
            n170 = call <vilib>:"Error Cluster From Error Code.vi"("show call chain? (False)"=TRUE, "error message (\"\")"=w359, "error code (0)"=1) -> ("error out"=w365:errorcluster)  [unwired: 6 in]
            n171 = Merge Errors(w366, w365) -> (w367:errorcluster)
          }
        }
        n172 = call-dynamic "Delacor_lib_QMH_Error Handler - Message Handling Loop.vi"("error in"=w194, "Message Queue in"=w185) -> ("dup error in"=w191:errorcluster)  [unwired: 8 in, 1 out]
      }
    }
    frame Error {
      n173 = call "Synchronize Caller Events.vi"("Module Admin"=w371) -> ("Module Admin out"=w370:refnum<class "Delacor_lib_QMH_Cloneable Module Admin.lvclass">)  [unwired: 9 in, 1 out]
      n174 = property on="Property Node" class="Mod Admin"(reference=w370) -> ("Accessors:Module ID"=w369:i32)  [unwired: 1 in, 2 out]
      n175 = call-dynamic "Delacor_lib_QMH_Release Message Queue.vi"("error in"=w377, "Message Queue"=w368) -> ("error out"=w376:errorcluster)  [unwired: 9 in]
      n176 = call "Module Name--constant.vi"("Module ID"=w369) -> ("Module Name"=w374:string)  [unwired: 10 in]
      n177 = Format Into String(format string="An error occurred during initialization. %s is no longer running.", w374) -> (resulting string=w372:string)  [unwired: 2 in, 1 out]
      n178 = call "Error Reported.vi"("Additional Information"=w372, "Error"=w376, "Module ID"=w369) -> ()  [unwired: 8 in, 1 out]
    }
  }
  n179 = Merge Errors(w17, w16) -> (w18:errorcluster)
  n180 = call "Close Module.vi"("error in"=w18, "Wait for stop?"=w2, "Module Admin in"=w4) -> ("error out"=w14:errorcluster, "External Launch"=w1:bool, "Module Admin out"=w3:refnum<class "Delacor_lib_QMH_Cloneable Module Admin.lvclass">)  [unwired: 6 in]
  n181 = Unregister For Events(event registration refnum=w9, error in=w14) -> (error out=w13:errorcluster)
  "error out" <- w13
  n182 = case "External Launch?" shown="True" w1 {
    tunnel: w13 -> [_ w378]
    frame False {
    }
    frame True {
      n183 = case shown="No Error" w378 {
        frame No Error {
          n184 = invoke class="VI" method="FP.Close"() -> ()  [unwired: 3 in, 3 out]
        }
        frame Error {
          n185 = disable-structure shown="Default" {
            frame condition #0 (active) {
              n186 = invoke class="VI" method="FP.Open"("Activate"=TRUE ("Activate?")) -> ()  [unwired: 4 in, 5 out]
            }
            frame condition #1 {
              # "Don't show panel on error if running inside a built EXE."
            }
          }
        }
      }
    }
  }
  n187 = local write "Module Admin"(w3) -> ()
